vi "Handle Last Ack Core.vi"(4 "error in (no error)":errorcluster, 6 "Last Ack":refnum<class "Last Ack.lvclass">, 7 "Form Server in":refnum<class "Form Server.lvclass">) -> (0 "error out":errorcluster, 3 "Form Server out":refnum<class "Form Server.lvclass">)   [LabVIEW 2020, in "Form Server.lvlib" / "Form Server.lvclass"]
doc: "(<B>Filename</B>: Actor Framework.lvlib:Actor.lvclass:Handle Last Ack Core.vi)\n\nDefines how the caller actor responds to the Last Ack message from a nested actor. The Last Ack message is the final message a nested actor sends to its caller before it shuts down. The message contains information about the final state of the nested actor.\n\nBy default, this method does nothing except return any error the nested actor sent. A descendant class may override this method to define behavior."
uses:
  Form Server.lvclass
  <vilib>/ActorFramework/LastAck/Last Ack.lvclass
  <vilib>/ActorFramework/LastAck/Last Ack.lvclass/Last Ack.ctl
  Form Model/Form Model.lvclass
  <vilib>/MGI/Monitored Actor/Monitored Actor/Monitored Actor/Monitored Actor.lvclass
  <vilib>/ActorFramework/Actor/Actor.lvclass
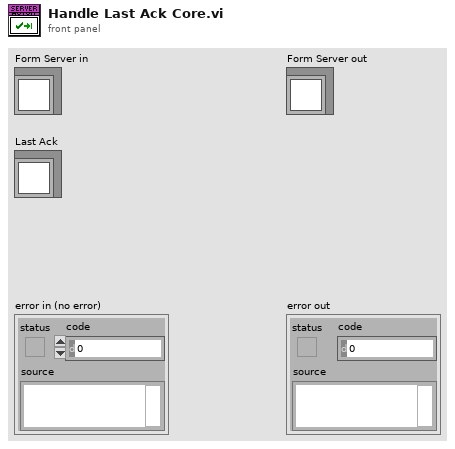
[diagram p1: front panel]
types:
  T1 = typedef "Form Server Interfaces.lvlib/Form ID.ctl" = cluster{"Name":string, "Panel type":string}
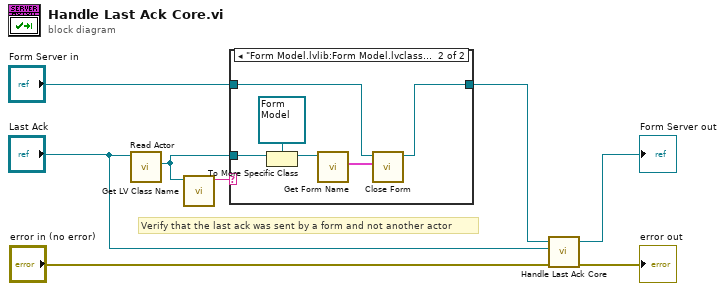
[diagram p0: block diagram]
diagram:
  # "Verify that the last ack was sent by a form and not another actor"
  n1 = call <vilib>:"Read Actor.vi"("Last Ack"="Last Ack") -> ("Actor"=w2:refnum<class "Actor.lvclass">)  [unwired: 10 in]
  n2 = call <vilib>:"Get LV Class Name.vi"("object"=w2) -> ("class name"=w1:string)  [unwired: 9 in, 1 out]
  n3 = case shown="\"Form Model.lvlib:Form Model.lvclass\"" w1 {
    tunnel: "Form Server in" -> [w9 w11]
    tunnel: [w9 w10] -> w4
    tunnel: w2 -> [_ w13]
    frame "", Default {
    }
    frame "Form Model.lvlib:Form Model.lvclass" {
      n4 = To More Specific Class(target class=refnum<class "Form Model.lvclass"> refnum ("Form Model.lvlib:Form Model.lvclass"), reference=w13) -> (specific class reference=w14:refnum<class "Form Model.lvclass">)  [unwired: 1 in, 1 out]
      n5 = call-dynamic "Get Form Name.vi"("Form Model in"=w14) -> ("Form ID"=w12:T1)  [unwired: 8 in, 2 out]
      n6 = call-dynamic "Close Form.vi"("Form Name"=w12, "Form Server in"=w11) -> ("Form Server out"=w10:refnum<class "Form Server.lvclass">)  [unwired: 8 in, 1 out]
    }
  }
  n7 = call-parent "Handle Last Ack Core.vi"("error in (no error)"="error in (no error)", "Last Ack"="Last Ack", "Actor in"=w4) -> ("error out"=→"error out":errorcluster, "Actor out"=→"Form Server out":refnum<class "Form Server.lvclass">)  [unwired: 3 in]
